vi "Control Sys Test.vi"() -> ()   [LabVIEW 2015]
uses:
  <vilib>/Platform/TimedLoop/XDataNode/timing_clust.ctl
  <vilib>/Platform/TimedLoop/XDataNode/nitl_modes.ctl
  <vilib>/Platform/TimedLoop/XDataNode/wakeup.ctl
  <vilib>/FPGAPlugInAG/myRIO-1900/niLvFpga_Open_myRIO-1900.vi
  <vilib>/rvi/interface/common/dynamic/niFpgaDynamicAddResources.vi
  <vilib>/myRIO/Common/Instrument Driver Framework/Utilities/vis/FPGA Ref Manager.vi
  <vilib>/Utility/error.llb/Error Cluster From Error Code.vi
  <vilib>/myRIO/Common/Instrument Driver Framework/Utilities/vis/Ref Counter.vi
  Localization/Right Variables.vi
  <vilib>/rvi/interface/nirviOpenFPGA/nirviOpenFPGA.xnode
  Localization/LidarLitev3test_FPGATarget_FPGAMainwLidarLi_c8ybSBS-918.lvbitx
  <vilib>/platform/TimedLoop/XDataNode/XDataNode.xnode
  <vilib>/myRIO/Instrument Drivers/Utilities/Utilities.lvlib
  <vilib>/Platform/TimedLoop/XDataNode/XDNodeRunTimeDep.lvlib
panel:
  out "Waveform Chart":u16(graph)
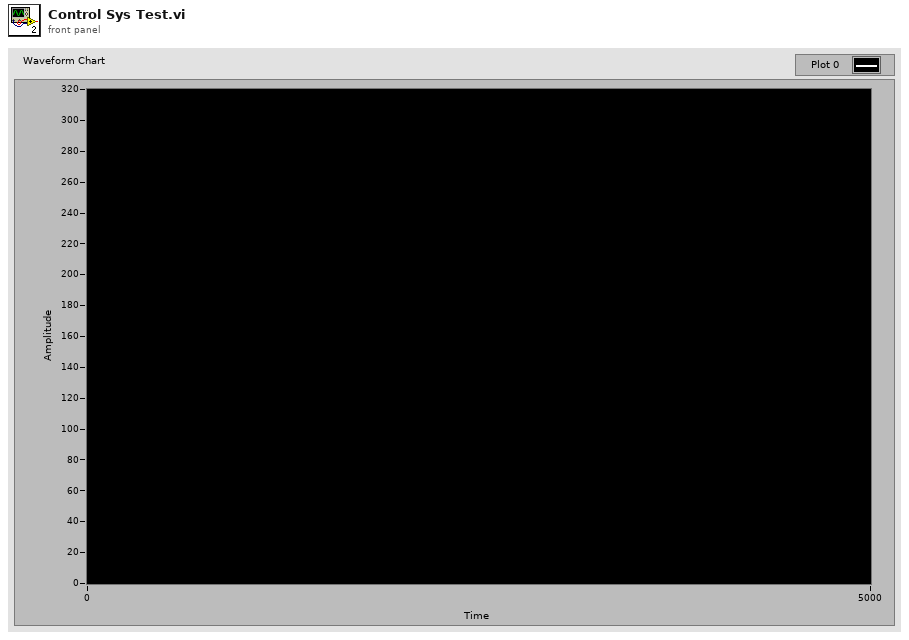
[diagram p1: front panel]
types:
  T1 = typedef "XDNodeRunTimeDep.lvlib/timing_clust.ctl" = cluster{"Expected End [f-1]":u64, "Actual End [f-1]":u64, "Finished Late? [f-1]":bool, "Expected End [i-1]":u64, "Actual End [i-1]":u64, "Finished Late? [i-1]":bool, "Expected Start [i]":u64, "Actual Start [i]":u64, "Expected Start [f]":u64, "Actual Start [f]":u64, "Source Name":string, "Structure Name":string, "Period":i64, "Deadline":i64, "Offset":i64, "Start":i64, "Priority":i32, "Timeout":i32, "Mode":T2, "Wakeup Reason":T3, "Error":errorcluster, "Source Type":string, "Secondary Source Type":string, "Global End Time":u64, "Global Start Time":u64, "Frame Duration":u64, "Iteration Duration":u64, "Assigned CPU":i32, "I/O Scan Engine Mode":u32}
  T2 = typedef "XDNodeRunTimeDep.lvlib/nitl_modes.ctl" = enum32{"No Change", "Process missed periods, maintain original phase", "Discard missed periods, maintain original phase", "Process missed periods, ignore original phase", "Discard missed periods, ignore original phase"}
  T3 = typedef "XDNodeRunTimeDep.lvlib/wakeup.ctl" = enum32{"Normal", "Aborted", "Asynchronous wakeup", "Timing source error", "Timed loop error", "Timeout"}
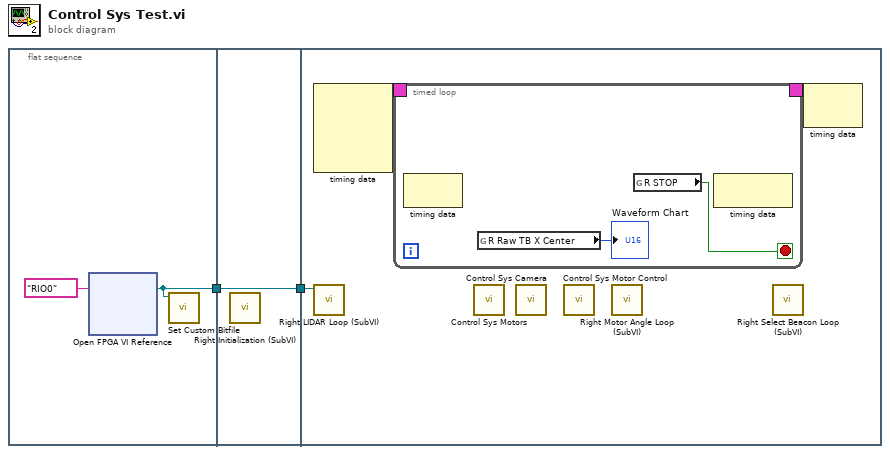
[diagram p0: block diagram]
diagram:
  n1 = flat-sequence {
    tunnel: [w4] -> w2
    tunnel: w2 -> [w5]
    tunnel: [w5] -> w1
    tunnel: w1 -> [w8]
    frame #0 {
      n2 = xnode "Open FPGA VI Reference"("resource name"=tag "RIO0") -> ("FPGA VI Reference Out"=w4:refnum<k20>)  [unwired: 1 in, 1 out]
      n3 = call <vilib>:"Set Custom Bitfile.vi"("Custom FPGA Reference In"=w4) -> ()  [unwired: 9 in, 2 out]
    }
    frame #1 {
      n4 = call "Right Initialization (SubVI).vi"() -> ()  [unwired: 12 in]
    }
    frame #2 {
      n5 = node-c288() -> (w7:T1)  [unwired: 4 in]
      n6 = call "Right LIDAR Loop (SubVI).vi"("Refnum in"=w8) -> ()  [unwired: 11 in]
      n7 = timed-loop {
        timing: w7 -> [_]
        timing-out: [_] -> w6
        stop <- w9 stop-if-true
        n8 = node-c288() -> ()  [unwired: 1 in, 1 out]
        n9 = global read "Right Variables.vi" "R Raw TB X Center"() -> (→"Waveform Chart":u16)
        n10 = global read "Right Variables.vi" "R STOP"() -> (w9:bool)
        n11 = node-c288() -> ()  [unwired: 1 in, 1 out]
      }
      n12 = call "Control Sys Motors.vi"() -> ()  [unwired: 12 in]
      n13 = call "Control Sys Camera.vi"() -> ()  [unwired: 12 in]
      n14 = call "Control Sys Motor Control.vi"() -> ()  [unwired: 12 in]
      n15 = call "Right Motor Angle Loop (SubVI).vi"() -> ()  [unwired: 12 in]
      n16 = call "Right Select Beacon Loop (SubVI).vi"() -> ()  [unwired: 12 in]
      n17 = node-c288(w6) -> ()  [unwired: 1 out]
    }
  }
